vi "WT_Single_Pass_analysis.vi"(0 "Displacement":dbl[](array[numeric]), 1 "Start Cut Deg":dbl, 2 "End Cut Deg":dbl, 3 "Radius":dbl=200.0) -> (4 "Blade Angles":dbl[](array[numeric]), 5 "Blade Positions":dbl[](array[numeric]), 6 "Blade1":dbl[](graph), 7 "Blade 2":dbl[](graph), 8 "Blade 3":dbl[](graph))   [LabVIEW 2022 SP3]
uses:
  <vilib>/Analysis/baseanly.llb/Mean (DBL).vi
  <vilib>/Analysis/NI_AALPro.lvlib
  <vilib>/Analysis/NI_AALBase.lvlib
panel:
  out "Disp in":dbl[](graph)
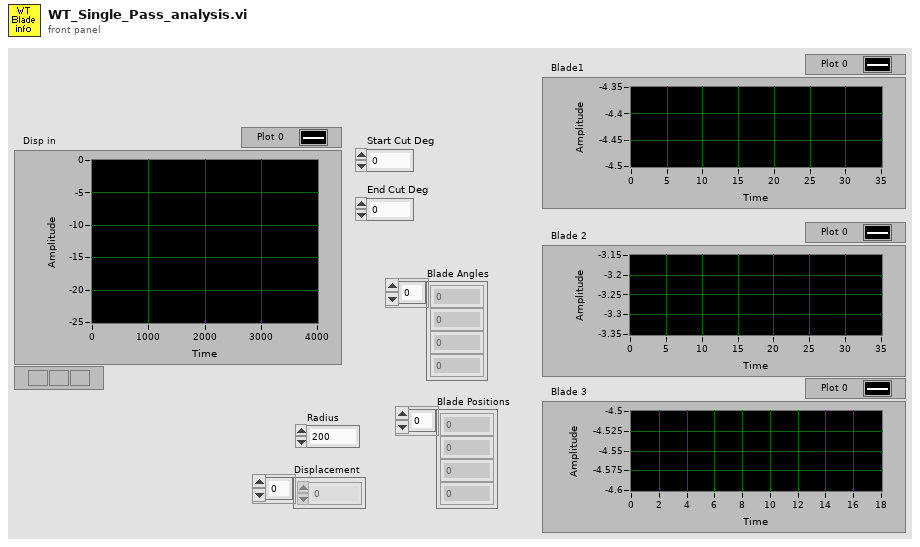
[diagram p1: front panel]
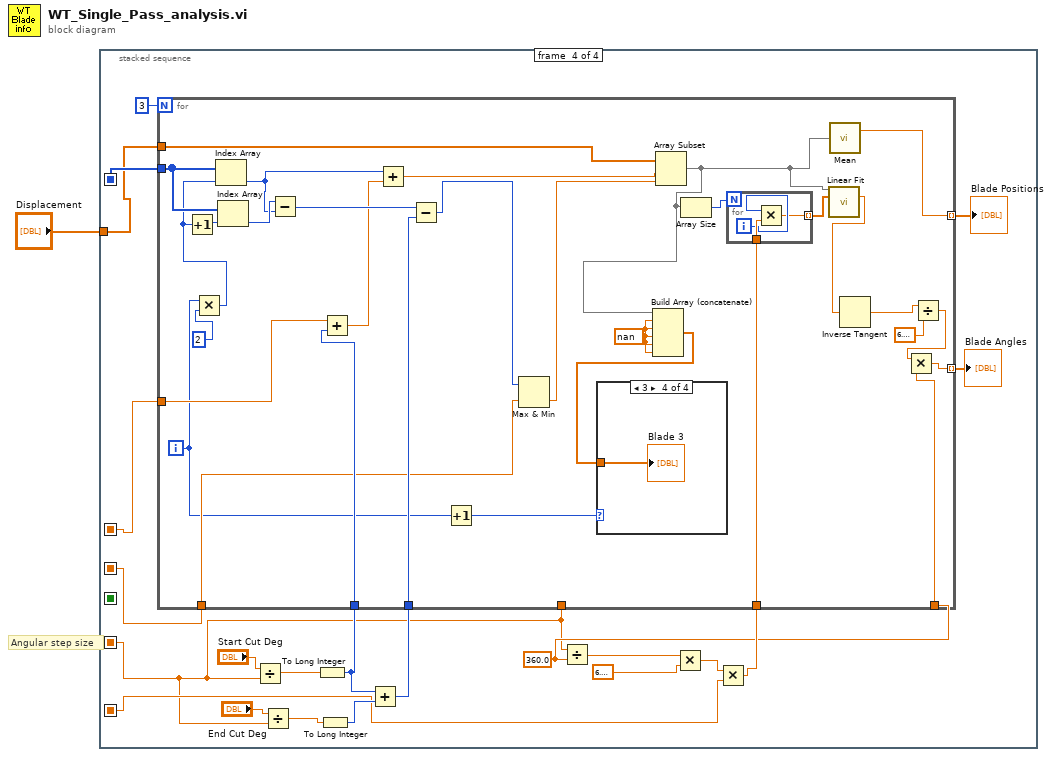
[diagram p0: block diagram]
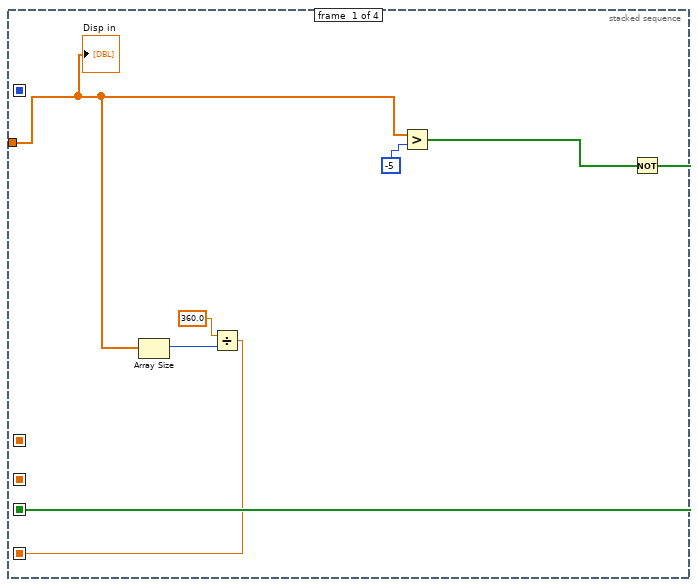
[diagram p2: hidden frame]
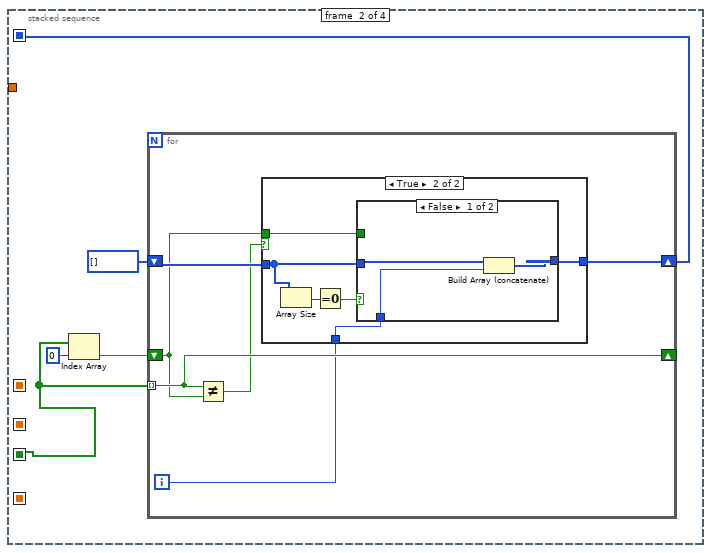
[diagram p3: hidden frame]
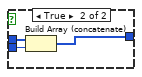
[diagram p6: hidden frame]
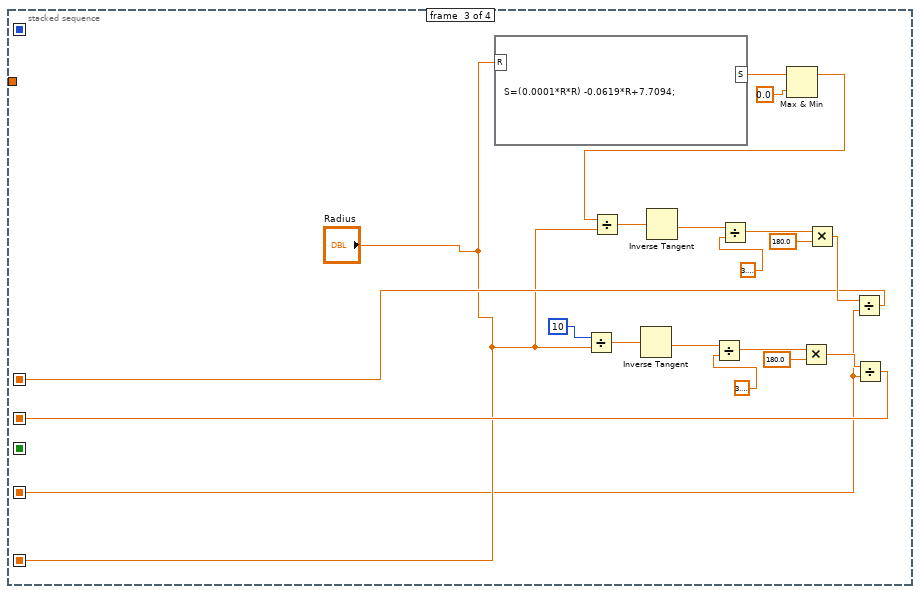
[diagram p7: hidden frame]
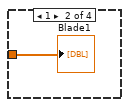
[diagram p9: hidden frame]
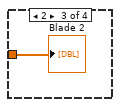
[diagram p10: hidden frame]
diagram:
  # "Angular step size"
  n1 = stacked-sequence {
    seq-local: [w8 _ _ _] -> [_ w9 _ _]
    seq-local: [_ w10 _ _] -> [_ _ _ w73]
    seq-local: [_ _ "Radius" _] -> [_ _ _ w64]
    seq-local: [_ _ w43 _] -> [_ _ _ w63]
    seq-local: [_ _ w45 _] -> [_ _ _ w62]
    seq-local: [w3 _ _ _] -> [_ _ w38 w58]
    tunnel: "Displacement" -> [w2 _ _ w61]
    frame #0 {
      n2 = Array Size(array=w2) -> (size(s)=w4:i32)
      n3 = Divide(x=360.0, y=w4) -> (x/y=w3:dbl)
      n4 = Greater?(x=w2, y=-5) -> (0:w6:bool[])
      n5 = Not(x=w6) -> (.not. x?=w8:bool[])
      "Disp in" <- w2
    }
    frame #1 {
      n6 = Index Array(array=w9, index=0) -> (element=w12:bool)
      n7 = for {
        tunnel: w9 -> [w19] mode=indexing
        shift-right: [w19] -> _
        shift-left: w12 -> [w14]
        shift-right: [w16] -> w10
        shift-left: i32[] [] -> [w17]
        i -> [w18]
        n8 = Not Equal?(x=w19, y=w14) -> (x != y?=w15:bool)
        n9 = case shown="True" w15 {
          tunnel: w18 -> [_ w26]
          tunnel: w17 -> [w20 w24]
          tunnel: [w20 w25] -> w16
          tunnel: w14 -> [_ w21]
          frame False {
          }
          frame True {
            n10 = Array Size(array=w24) -> (size(s)=w23:i32)
            n11 = Equal To 0?(x=w23) -> (x = 0?=w22:bool)
            n12 = case shown="False" w22 {
              tunnel: w26 -> [w27 w33]
              tunnel: w24 -> [w29 w32]
              tunnel: [w28 w31] -> w25
              tunnel: w21 -> [_ w30]
              frame False {
                n13 = Build Array (concatenate)(w29, w27) -> (w28:i32[])
              }
              frame True {
                n14 = case shown="False" w30 {
                  tunnel: w33 -> [_ w37]
                  tunnel: w32 -> [w34 w36]
                  tunnel: [w34 w35] -> w31
                  frame False {
                  }
                  frame True {
                    n15 = Build Array (concatenate)(w36, w37) -> (w35:i32[])
                  }
                }
              }
            }
          }
        }
      }
    }
    frame #2 {
      n16 = formula code="S=(0.0001*R*R) -0.0619*R+7.7094;"("R"="Radius") -> ("S"=w42:dbl)
      n17 = Divide(x=10, y="Radius") -> (x/y=w56:dbl)
      n18 = Inverse Tangent(1:w56) -> (0:w55:dbl)
      n19 = Divide(x=w55, y=3.141592653589793) -> (x/y=w53:dbl)
      n20 = Max & Min(x=w42, y=0.0) -> (max(x,y)=w40:dbl)  [unwired: 1 out]
      n21 = Divide(x=w40, y="Radius") -> (x/y=w47:dbl)
      n22 = Inverse Tangent(1:w47) -> (0:w48:dbl)
      n23 = Divide(x=w48, y=3.141592653589793) -> (x/y=w50:dbl)
      n24 = Multiply(x=w53, y=180.0) -> (x*y=w44:dbl)
      n25 = Multiply(x=w50, y=180.0) -> (x*y=w46:dbl)
      n26 = Divide(x=w46, y=w38) -> (x/y=w45:dbl)
      n27 = Divide(x=w44, y=w38) -> (x/y=w43:dbl)
    }
    frame #3 {
      w65 = 360.0 ("y")
      n28 = Divide(x="Start Cut Deg", y=w58) -> (x/y=w75:dbl)
      n29 = Divide(x="End Cut Deg", y=w58) -> (x/y=w76:dbl)
      n30 = To Long Integer(number=w75) -> (32bit integer=w71:i32)
      n31 = To Long Integer(number=w76) -> (32bit integer=w74:i32)
      n32 = Add(x=w71, y=w74) -> (x+y=w70:i32)
      n33 = Divide(x=w58, y=w65) -> (x/y=w69:dbl)
      n34 = Multiply(x=w69, y=6.283185307179586) -> (x*y=w68:dbl)
      n35 = Multiply(x=w68, y=w64) -> (x*y=w66:dbl)
      n36 = for {
        N: 3 -> [_]
        tunnel: w61 -> [w106]
        tunnel: w73 -> [w103]
        tunnel: w71 -> [w92]
        tunnel: w70 -> [w99]
        tunnel: w66 -> [w98]
        tunnel: w65 -> [w93]
        tunnel: w58 -> [_]
        tunnel: w63 -> [w85]
        tunnel: w62 -> [w90]
        tunnel: [w88] -> w60 mode=indexing
        tunnel: [w87] -> w59 mode=indexing
        i -> [w83]
        w79 = nan
        n37 = Multiply(x=w83, y=2) -> (x*y=w101:i32)
        n38 = Increment(x=w101) -> (x+1=w100:i32)
        n39 = Index Array(array=w103, index=w101) -> (element=w108:i32)
        n40 = Index Array(array=w103, index=w100) -> (element=w109:i32)
        n41 = Subtract(x=w109, y=w108) -> (x-y=w107:i32)
        n42 = Add(x=w90, y=w92) -> (x+y=w91:dbl)
        n43 = Add(x=w108, y=w91) -> (x+y=w89:dbl)
        n44 = Subtract(x=w107, y=w99) -> (x-y=w86:i32)
        n45 = Increment(x=w83) -> (x+1=w82:i32)
        n46 = Max & Min(x=w86, y=w85) -> (min(x,y)=w84:dbl)  [unwired: 1 out]
        n47 = Array Subset(array=w106, index=w89, length=w84) -> (w81:dbl[])
        n48 = Build Array (concatenate)(w81, w79, w79, w79, w79, w79) -> (w80:dbl[])
        n49 = case shown="3" w82 {
          tunnel: w80 -> [_ w110 w111 w112]
          frame 0, Default {
          }
          frame 1 {
            "Blade1" <- w110
          }
          frame 2 {
            "Blade 2" <- w111
          }
          frame 3 {
            "Blade 3" <- w112
          }
        }
        n50 = Array Size(array=w81) -> (size(s)=w105:i32)
        n51 = for {
          N: w105 -> [_]
          tunnel: w98 -> [w115]
          tunnel: [w113] -> w104 mode=indexing
          i -> [w114]
          n52 = Multiply(x=w114, y=w115) -> (x*y=w113:dbl)
        }
        n53 = call <vilib>:"Linear Fit.vi"("Y"=w81, "X"=w104) -> ("slope"=w97:dbl)  [unwired: 9 in, 4 out]
        n54 = call-poly <vilib>:"Mean.vi"("X"=w81) -> ("mean"=w87:dbl)  [unwired: 1 out]
        n55 = Inverse Tangent(1:w97) -> (0:w96:dbl)
        n56 = Divide(x=w96, y=6.283185307179586) -> (x/y=w94:dbl)
        n57 = Multiply(x=w94, y=w93) -> (x*y=w88:dbl)
      }
      "Blade Angles" <- w60
      "Blade Positions" <- w59
    }
  }
